vi "SpikeEdit.vi"(1 "tolerance":dbl format="%.2f", 2 "column":u8, 3 "data in":dbl[][](array[numeric]) format="%.2f") -> (0 "data out":dbl[][](array[numeric]) format="%.2f")   [LabVIEW 2018]
uses:
  <vilib>/Analysis/NI_AALBase.lvlib
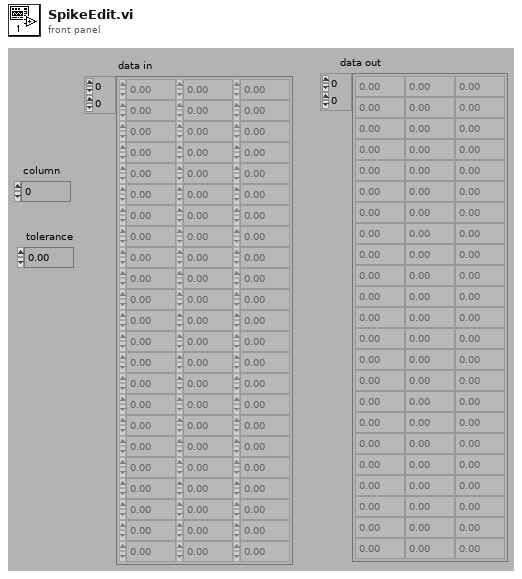
[diagram p1: front panel]
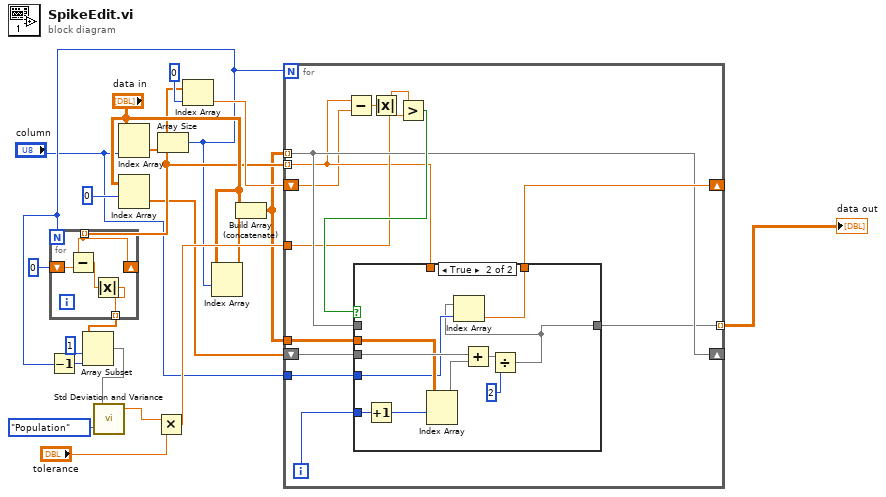
[diagram p0: block diagram]
diagram:
  n1 = Index Array(array="data in", index (col)="column") -> (element=w9:dbl[])  [unwired: 1 in]
  n2 = Index Array(array="data in", index (row)=0) -> (element=w6:dbl[])  [unwired: 1 in]
  n3 = Array Size(array=w9) -> (size(s)=w8:i32)
  n4 = Decrement(x=w8) -> (x-1=w19:i32)
  n5 = for {
    N: w8 -> [_]
    shift-right: [w23] -> _
    shift-left: 0 -> [w24]
    tunnel: w9 -> [w23] mode=indexing
    tunnel: [w21] -> w17 mode=indexing
    n6 = Subtract(x=w23, y=w24) -> (x-y=w22:dbl)
    n7 = Absolute Value(x=w22) -> (abs(x)=w21:dbl)
  }
  n8 = Array Subset(array=w17, index=1, length=w19) -> (w3:dbl[])
  n9 = call <vilib>:"Std Deviation and Variance.vi"("X"=w3, "Weighting (Sample)"=enum16{"Sample", "Population"}."Population") -> ("mean"=w12:dbl)  [unwired: 2 out]
  n10 = Multiply(x=w12, y="tolerance") -> (x*y=w14:dbl)
  n11 = Index Array(array=w9, index=0) -> (element=w16:dbl)
  n12 = Index Array(array="data in", index (row)=w8) -> (element=w13:dbl[])  [unwired: 1 in]
  n13 = Build Array (concatenate)("data in", w13) -> (w5:dbl[][])
  n14 = for {
    N: w8 -> [_]
    tunnel: w9 -> [w27] mode=indexing
    shift-right: [w33] -> _
    shift-left: w16 -> [w26]
    tunnel: w14 -> [w28]
    tunnel: w5 -> [w31] mode=indexing
    shift-right: [w31] -> _
    shift-left: w6 -> [w32]
    tunnel: w5 -> [w30]
    tunnel: [w29] -> w4 mode=indexing
    tunnel: "column" -> [w25]
    i -> [w35]
    n15 = Subtract(x=w27, y=w26) -> (x-y=w37:dbl)
    n16 = Absolute Value(x=w37) -> (abs(x)=w36:dbl)
    n17 = Greater?(x=w36, y=w28) -> (0:w34:bool)
    n18 = case shown="True" w34 {
      tunnel: [w38 w40] -> w29
      tunnel: w35 -> [_ w48]
      tunnel: [w39 w42] -> w33
      tunnel: w27 -> [w39 _]
      tunnel: w31 -> [w38 _]
      tunnel: w32 -> [_ w46]
      tunnel: w30 -> [_ w45]
      tunnel: w25 -> [_ w41]
      frame False {
      }
      frame True {
        n19 = Increment(x=w48) -> (x+1=w49:i32)
        n20 = Index Array(array=w45, index (row)=w49) -> (element=w47:dbl[])  [unwired: 1 in]
        n21 = Add(x=w46, y=w47) -> (x+y=w44:dbl[])
        n22 = Divide(x=w44, y=2) -> (x/y=w40:dbl[])
        n23 = Index Array(array=w40, index=w41) -> (element=w42:dbl)
      }
    }
  }
  "data out" <- w4
